vi "Do.vi"(8 "error in (no error)":errorcluster, 10 "Actor in":refnum<class "Actor.lvclass">, 11 "Update Connection State Msg":refnum<class "Update Connection State Msg.lvclass">) -> (0 "error out":errorcluster, 2 "Actor out":refnum<class "Actor.lvclass">)   [LabVIEW 2014, in "GoBang.lvlib" / "Update Connection State Msg.lvclass"]
doc: "This VI delivers the message to the actor by calling the appropriate method(s) on the actor."
uses:
  Update Connection State Msg.lvclass
  <vilib>/ActorFramework/Actor/Actor.lvclass
  Server/CS++GoBangServer.lvclass
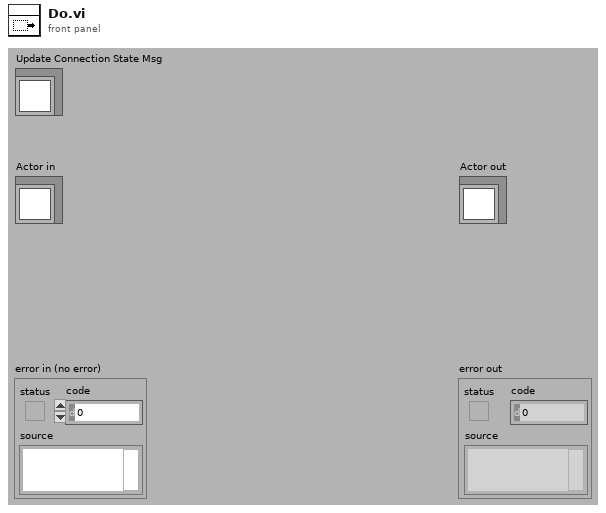
[diagram p1: front panel]
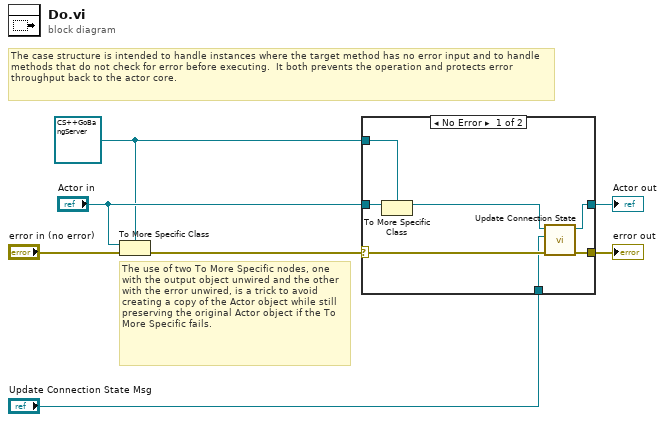
[diagram p0: block diagram]
diagram:
  w2 = refnum<class "CS++GoBangServer.lvclass"> refnum ("Actor in")
  # "The use of two To More Specific nodes, one with the output object unwired and the other with the error unwired, is a trick to avoid creating a copy of the Actor object while still preserving the original Actor object if the To More Specific fails."
  # "The case structure is intended to handle instances where the target method has no error input and to handle methods that do not check for error before executing.  It both prevents the operation and protects error throughput back to the actor core."
  n1 = To More Specific Class(target class=w2, reference="Actor in", error in="error in (no error)") -> (error out=w6:errorcluster)  [unwired: 1 out]
  n2 = case shown="No Error" w6 {
    selector: w6 -> [w12 w16]
    tunnel: [w14 w16] -> w5
    tunnel: [w13 w15] -> w4
    tunnel: "Actor in" -> [w11 w15]
    tunnel: w2 -> [w10 _]
    tunnel: "Update Connection State Msg" -> [w8 _]
    frame No Error {
      n3 = To More Specific Class(target class=w10, reference=w11) -> (specific class reference=w9:refnum<class "CS++GoBangServer.lvclass">)  [unwired: 1 in, 1 out]
      n4 = call-dynamic "Update Connection State.vi"("error in (no error)"=w12, "Update Connection State Msg"=w8, "CS++GoBangServer in"=w9) -> ("error out"=w14:errorcluster, "CS++GoBangServer out"=w13:refnum<class "CS++GoBangServer.lvclass">)  [unwired: 7 in]
    }
    frame Error {
      # "If type check fails, pass the original object out again."
    }
  }
  "error out" <- w5
  "Actor out" <- w4
